vi "9217_Channels to Config.vi"(8 "error in (no error)":errorcluster, 10 "Conversion Time":u16(ring) items=["200 ms", "2.5 ms"], 11 "Channels":T1(array[cluster])) -> (0 "error out":errorcluster, 3 "_9217 Config Data":T2={"Conversion Time"=0, "Degree Range"=[], "RTD_Type"=[1], "RTD_A"=[], "RTD_B"=[], "RTD_C"=[], "RTD_Ro"=[]} {"Conversion Time" items=["200 ms", "2.5 ms"]; "Degree Range" items=["Raw Ohms", "Degrees Kelvin", "Degrees Celsius", "Degrees Fahrenheit", "Degrees Rankine"]; "RTD_Type" items=["TCR3851"=1, "TCR3750"=2, "TCR3916"=3, "TCR3920"=4, "TCR3911"=5, "TCR3928"=6, "Custom"=0]})   [LabVIEW 2011, in "Modules.lvlib" / "9217.lvclass"]
uses:
  9217.lvclass
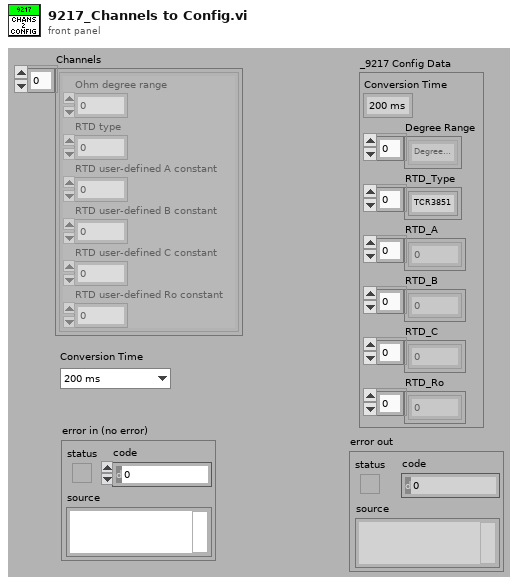
[diagram p1: front panel]
types:
  T1 = cluster{"Ohm degree range":u32, "RTD type":u32, "RTD user-defined A constant":dbl, "RTD user-defined B constant":dbl, "RTD user-defined C constant":dbl, "RTD user-defined Ro constant":dbl}[]
  T2 = cluster{"Conversion Time":u16, "Degree Range":u8[], "RTD_Type":u8[], "RTD_A":dbl[], "RTD_B":dbl[], "RTD_C":dbl[], "RTD_Ro":dbl[]}
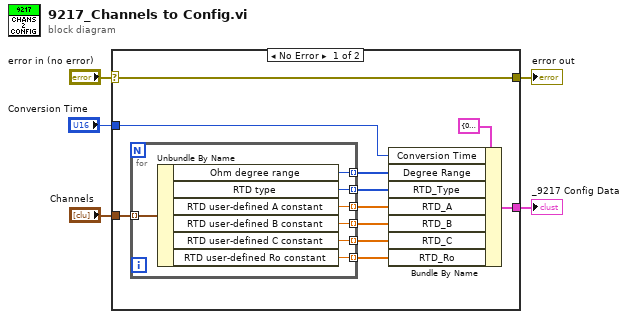
[diagram p0: block diagram]
diagram:
  n1 = case shown="No Error" "error in (no error)" {
    selector: "error in (no error)" -> [w6 w24]
    tunnel: [w6 w24] -> w4
    tunnel: "Channels" -> [w15 _]
    tunnel: "Conversion Time" -> [w14 _]
    tunnel: [w7 _] -> w1
    frame No Error {
      n2 = for {
        tunnel: w15 -> [w23] mode=indexing
        tunnel: [w22] -> w13 mode=indexing
        tunnel: [w21] -> w12 mode=indexing
        tunnel: [w20] -> w11 mode=indexing
        tunnel: [w19] -> w10 mode=indexing
        tunnel: [w18] -> w9 mode=indexing
        tunnel: [w17] -> w8 mode=indexing
        n3 = Unbundle By Name(w23) -> ("Ohm degree range"=w22:u32, "RTD type"=w21:u32, "RTD user-defined A constant"=w20:dbl, "RTD user-defined B constant"=w19:dbl, "RTD user-defined C constant"=w18:dbl, "RTD user-defined Ro constant"=w17:dbl)
      }
      n4 = Bundle By Name(cluster=T2 {"Conversion Time"=0, "Degree Range"=[], "RTD_Type"=[1], "RTD_A"=[], "RTD_B"=[], "RTD_C"=[], "RTD_Ro"=[]} ("_9217 Config Data"), "Conversion Time"=w14, "Degree Range"=w13, "RTD_Type"=w12, "RTD_A"=w11, "RTD_B"=w10, "RTD_C"=w9, "RTD_Ro"=w8) -> (w7:T2)
    }
    frame Error {
    }
  }
  "_9217 Config Data" <- w1
  "error out" <- w4
